vi "SaveCsvDATE.vi"() -> (2 "结果字符串":string)   [LabVIEW 2018]
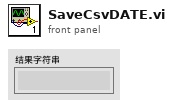
[diagram p1: front panel]
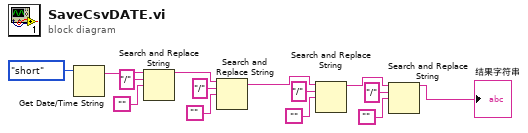
[diagram p0: block diagram]
diagram:
  n1 = Get Date/Time String(date format (0)=enum16{"short", "long", "abbreviated"}."short" ("日期格式(0)")) -> (date string=w13:string)  [unwired: 2 in, 1 out]
  n2 = Search and Replace String(input string=w13, search string="/" ("搜索字符串"), replace string="") -> (result string=w8:string)  [unwired: 5 in, 3 out]
  n3 = Search and Replace String(input string=w8, search string="/" ("搜索字符串"), replace string="") -> (result string=w2:string)  [unwired: 5 in, 3 out]
  n4 = Search and Replace String(input string=w2, search string="/" ("搜索字符串"), replace string="") -> (result string=w3:string)  [unwired: 5 in, 3 out]
  n5 = Search and Replace String(input string=w3, search string="/" ("搜索字符串"), replace string="") -> (result string=→"结果字符串":string)  [unwired: 5 in, 3 out]
